vi "Enqueue Multiple Commands (Array).vi"(8 "Error In":errorcluster, 10 "Commands' Data (Default = Empty)":variant[](array[variant]), 11 "Commands":T1[](array[typedef])) -> (0 "Error Out":errorcluster)   [LabVIEW 2023, in "Error Manager.lvlib" / "New Error Window.lvlib" / "MHL Queue.lvlib"]
doc: "Issues multiple commands by enqueuing multiple messages into the module's command queue. The commands should be received by calling the 'Dequeue' VI."
uses:
  MHL Queue.lvlib
  Command (enum).ctl
panel:
  # "Input\nInputs to the VI"
  # "Development\nControls or indicators that are useful for development or testing, but which are not outputs of the VI."
  # "Output\nOutputs of the VI"
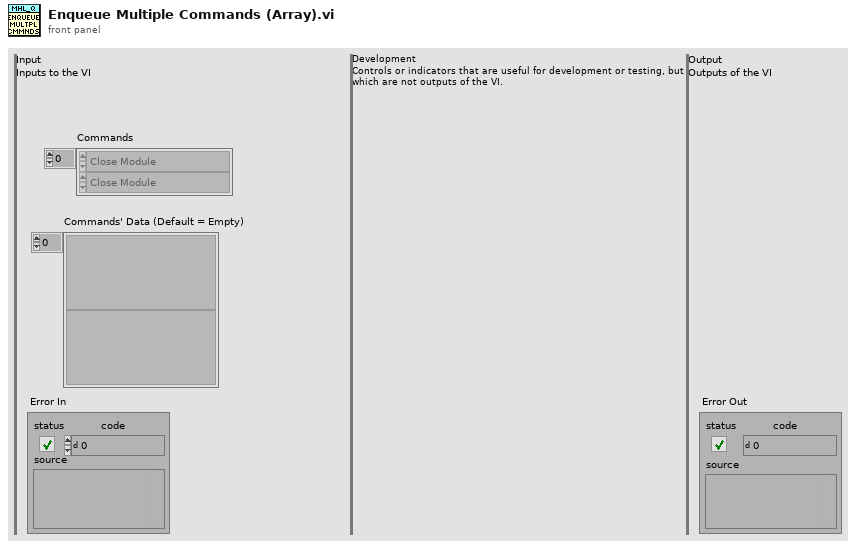
[diagram p1: front panel]
types:
  T1 = typedef "Error Manager.lvlib/New Error Window.lvlib/MHL Queue.lvlib/Command (enum).ctl" = enum16{"Init Module", "Close Module", "Handle Local Error", "OK Button Pressed"}
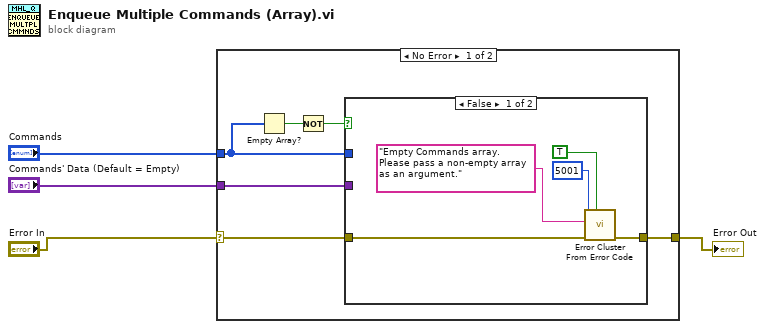
[diagram p0: block diagram]
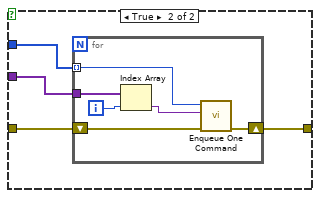
[diagram p2: hidden frame]
diagram:
  n1 = case shown="No Error" "Error In" {
    selector: "Error In" -> [w10 w26]
    tunnel: [w9 w26] -> w3
    tunnel: "Commands" -> [w6 _]
    tunnel: "Commands' Data (Default = Empty)" -> [w5 _]
    frame No Error {
      n2 = Empty Array?(array=w6) -> (empty?=w8:bool)
      n3 = Not(x=w8) -> (.not. x?=w7:bool)
      n4 = case shown="False" w7 {
        tunnel: [w14 w18] -> w9
        tunnel: w10 -> [w15 w19]
        tunnel: w6 -> [_ w17]
        tunnel: w5 -> [_ w16]
        frame False {
          n5 = call <vilib>:"Error Cluster From Error Code.vi"("show call chain? (False)"=TRUE, "error in (no error)"=w15, "error message (\"\")"="Empty Commands array. Please pass a non-empty array as an argument.", "error code (0)"=5001) -> ("error out"=w14:errorcluster)  [unwired: 5 in]
        }
        frame True {
          n6 = for {
            shift-right: [w24] -> w18
            shift-left: w19 -> [w25]
            tunnel: w17 -> [w23] mode=indexing
            tunnel: w16 -> [w22]
            i -> [w21]
            n7 = Index Array(array=w22, index=w21) -> (element=w20:variant)
            n8 = call "Enqueue One Command.vi"("error in (no error)"=w25, "Data"=w20, "Command"=w23) -> ("error out"=w24:errorcluster)  [unwired: 8 in]
          }
        }
      }
    }
    frame Error {
    }
  }
  "Error Out" <- w3
